vi "StringToBitArray.vi"(10 "string":string) -> (2 "Array":bool[](array[boolean]))   [LabVIEW 2016]
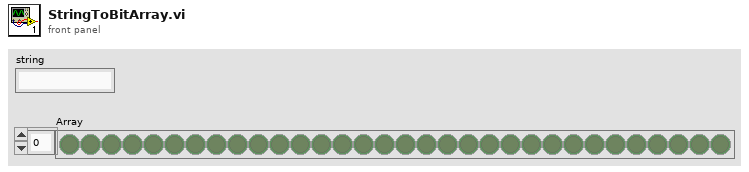
[diagram p1: front panel]
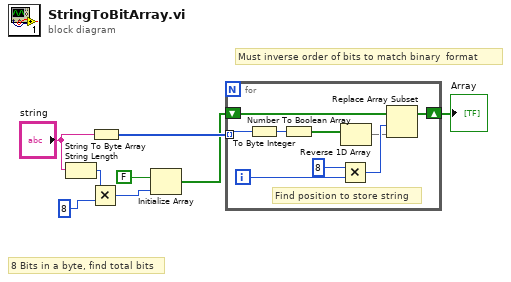
[diagram p0: block diagram]
diagram:
  # "8 Bits in a byte, find total bits"
  # "Must inverse order of bits to match binary  format"
  n1 = String Length(string="string") -> (length=w4:i32)
  n2 = Multiply(x=w4, y=8) -> (x*y=w2:i32)
  n3 = String To Byte Array(string="string") -> (unsigned byte array=w8:u8[])
  n4 = Initialize Array(FALSE, w2) -> (w6:bool[])
  n5 = for {
    tunnel: w8 -> [w12] mode=indexing
    shift-right: [w17] -> w5
    shift-left: w6 -> [w11]
    i -> [w16]
    # "Find position to store string"
    n6 = To Byte Integer(number=w12) -> (8bit integer=w13:i8)
    n7 = Number To Boolean Array(number=w13) -> (Boolean array=w10:bool[])
    n8 = Multiply(x=8, y=w16) -> (x*y=w14:i32)
    n9 = Reverse 1D Array(array=w10) -> (reversed array=w9:bool[])
    n10 = Replace Array Subset(array=w11, new element=w9, index=w14) -> (w17:bool[])
  }
  "Array" <- w5
